vi "LinkamStageController.vi"() -> ()   [LabVIEW 2013]
doc: "The Grab and Save to AVI VI acquires images continuously using the high-level acquisition VIs, displays them in an image control, and saves the images to an AVI file. A grab is appropriate for high-speed applications that process only one image at a time. Use an AVI file to save multiple images to a single file for post-processing or record images.\n\nIMAQ Init initializes the device. IMAQ Grab Setup initializes the grab function and starts capturing images to an internal software buffer. IMAQ Create creates an image buffer IMAQ Grab Acquire copies the internal buffer to Image out, and an image control displays the image on the front panel. IMAQ Close releases resources associated with the acquisition, and IMAQ Dispose frees the image buffer.\n\nIMAQ AVI Create initializes the AVI file, IMAQ AVI WriteFrame adds each image to the AVI file, and IMAQ AVI Close completes writing to the AVI file. Call IMAQ AVI Create for each AVI file created."
uses:
  <vilib>/userdefined/High Color/IMAQdx.ctl
  Mag.ctl
  <vilib>/Instr/_visa.llb/VISA Open Access Mode.ctl
  ImageEnum4GFV.ctl
  RampProgramModel/RampProgramModel.lvclass
  AVI recoder state.ctl
  <vilib>/vision/Avi.llb/IMAQ AVI2 Refnum.ctl
  DateandTime.ctl
  RampProgramModel/RampProgramModel.lvclass/RampProgramModel.ctl
  TextOnImage.ctl
  Ascii Experiment Data.ctl
  RampState.ctl
  <vilib>/Instr/_visa.llb/VISA Configure Serial Port (Instr).vi
  <vilib>/Utility/file.llb/Read From Spreadsheet File (DBL).vi
  <vilib>/Utility/file.llb/Write To Spreadsheet File (string).vi
  <vilib>/vision/driver/NI_Vision_Acquisition_Software.lvlib
  <resource>/objmgr/imaqdx.rc
panel:
  in  "Max(µm)":dbl=55.0 min=0.0 format="%#_g µm"
  in  "Min(µm)":dbl=35.0 min=0.0 format="%#_g µm"
  in  "Enable Droplet Detection":bool=TRUE
  in  "Stop Recording\n@ Temp (°C)":dbl=5.0 format="%#_g °C"
  in  "Start Recording\n@ Temp (°C)":dbl=-2.0 format="%#_g °C"
  in  "Enable\nAutomatic\nRecording":bool=TRUE
  in  "Gain (0-570)":dbl=300.0 min=0.0 max=570.0 step=1.0
  in  "Shutter (1-4095)":dbl=4095.0 min=1.0 max=4095.0 step=1.0
  in  "High Resolution":bool
  in  "Remarks":string
  out "Goal":string
  out "Experiment Name":string
  in  "NewExperiment":bool
  out "File Path":path=path "E:/LINKAM Measurements_Naama"
  in  "Mag":T1
  out "Temp Chart":dbl(graph)
  out "Time Remaining\n(HH:MM:SS)":dbl format="%<%H:%M:%S>t"
  out "Ramp Program Table":string[][](table)
  in  "Clear Table":bool
  in  "Add Entry":bool
  in  "StopProgram":bool
  in  "RunProgram":bool
  in  "PauseProgram":bool
  in  "SaveProgram":bool
  in  "LoadProgram":bool
  in  "Cycles":u32=1 min=1 max=1000 step=1
  out "Cycle No.":u32=1 min=1 max=1000 step=1
  in  "Pump Speed":u8(slide) max=30 step=1 scale=0.0..30.0
  in  "DelayInComm(ms)":u32=50
  out "Video Grabber":bool
  out "Linkam Controller":bool
  out "Ramp Controller":bool
  out "Video Recorder":bool
  in  "Pause":bool caption="Start Cooling/Heating"
  in  "Stop":bool caption="Start Cooling/Heating"
  in  "Record":bool caption="Start Cooling/Heating"
  out "Status":string="Stop"
  in  "TakeRefImage":bool caption="Start Cooling/Heating"
  in  "Time Between Consecutive Frames (sec)":dbl=1.0 caption="Time Between \nConsecutive \nFrames (sec)" min=0.0 max=3600.0 step=0.01 format="%.2g s"
  out "Full avi Path and Name":path=path "Z:/Downloads/data/Test-18_05_2014-15_02_54.avi"
  out "Codec Type":string="Motion JPEG (NI Vision)"
  in  "index 2":i32=4
  in  "error in (no error) 2":errorcluster
  out "Status":string="Stopped"
  out "Repeat Program ind":u32=1 min=1 max=1000 step=1
  in  "error in (no error)":errorcluster
  out "Reference Image":T2(plugin-control)
  in  "Hold Cooling/Heating":bool caption="Start Cooling/Heating"
  in  "Stop Cooling/Heating":bool caption="Start Cooling/Heating"
  in  "Start Cooling/Heating":bool
  in  "Setpoint (°C)":dbl=28.0 min=-100.0 max=50.0 step=0.1 format="%.1g °C"
  in  "Cooling Rate (°C/min)":dbl=1.0 min=0.0 max=20.0 step=0.01 format="%.2g °C/min"
  out "Current Temp (°C)":dbl format="%.1g °C"
  out "Status of Liquied Nitrogen Pump":string="96"
  in  "Max Speed":bool
  in  "LNP mode":bool=TRUE
  out "Error Message":string
  out "Status of Temperature Controller":string
  out "Temp String (C)":string="0.0"
  out "Timer":u32=1002
  out "remaining string":string
  out "read buffer":string
  out "return count":u32
  in  "Session In":T3="cam0"
  out "Image":T2(plugin-control)
  in  "stop":bool
  # "Live Image"
  # "Reference Image"
  # "Select your Camera above"
  # "Linkam Temperature Controller"
  # "Experiment Data"
  # "Video Recorder"
  # "Engines Status"
  # "Status"
  # "Liquid Nitrogen Pump Controller"
  # "Pump Speed"
  # "Video Grabber"
  # "Error Message"
  # "Ramp Table Controller"
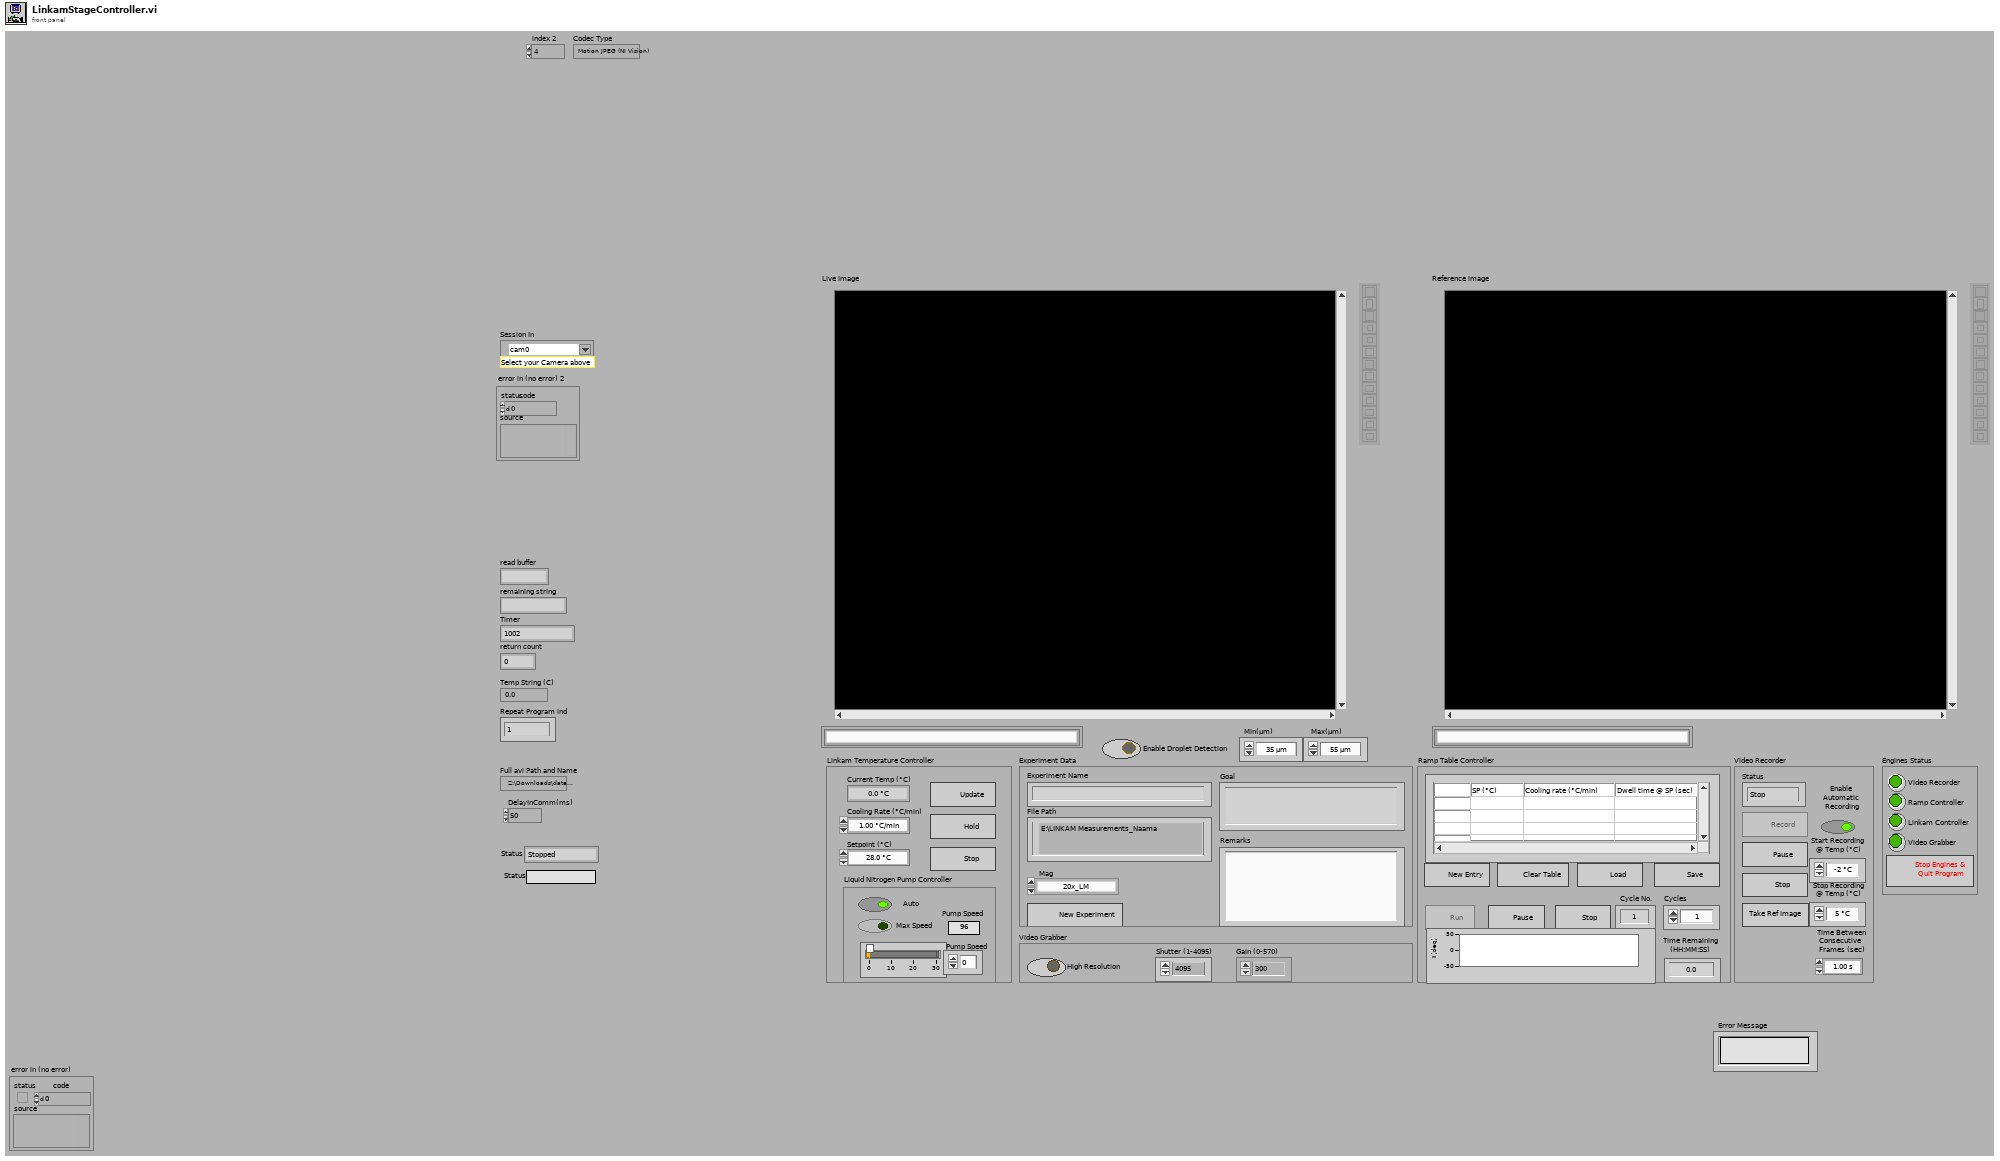
[diagram p1: front panel]
types:
  T1 = typedef "Mag.ctl" = enum16{"20x_LM", "50x_S", "100x_im"}
  T2 = typedef "IMAQ Image.ctl" = refnum<image>
  T3 = typedef "IMAQdx.ctl" = refnum<k21>
  T4 = enum8{"Enabled", "Disabled", "Disabled and Grayed Out"}
  T5 = typedef "DateandTime.ctl" = cluster{"Date and Time":string, "Temp (deg)":string}[]
  T6 = typedef "IMAQ AVI2 Refnum.ctl" = refnum<k20>
  T7 = typedef "AVI recoder state.ctl" = enum16{"Record", "Pause", "Stop", "Init"}
  T8 = typedef "ImageEnum4GFV.ctl" = enum16{"Delete", "Write", "Read", "Init"}
  T9 = typedef "VISA Open Access Mode.ctl" = u32
  T10 = typedef "RampState.ctl" = enum16{"Pause Program", "Heatling/Cooling", "Dwelling @ SP", "Stopped"}
  T11 = typedef "Ascii Experiment Data.ctl" = cluster{"Experiment Name":string, "Goal":string, "Remarks":string, "File Path":string, "Mag":string, "Repeat Program Number":string, "Full avi Path and Name":path, "Ramp Table ":string[][], "Date and Time":T5}
  T12 = cluster{"date/time string":string, "Temp String (C)":string}
  T13 = typedef "TextOnImage.ctl" = cluster{"Status":string, "Experiment Name":string, "Current Temp (C)":string, "Set Point (C)":string, "Cooling Rate (C/min)":string, "Mag":T1}
  T14 = cluster{"Position":cluster{"x":sgl, "y":sgl}, "Angle":sgl, "Scale":sgl, "Score":sgl, "Bounding Box":cluster{"x":sgl, "y":sgl}[]}[]
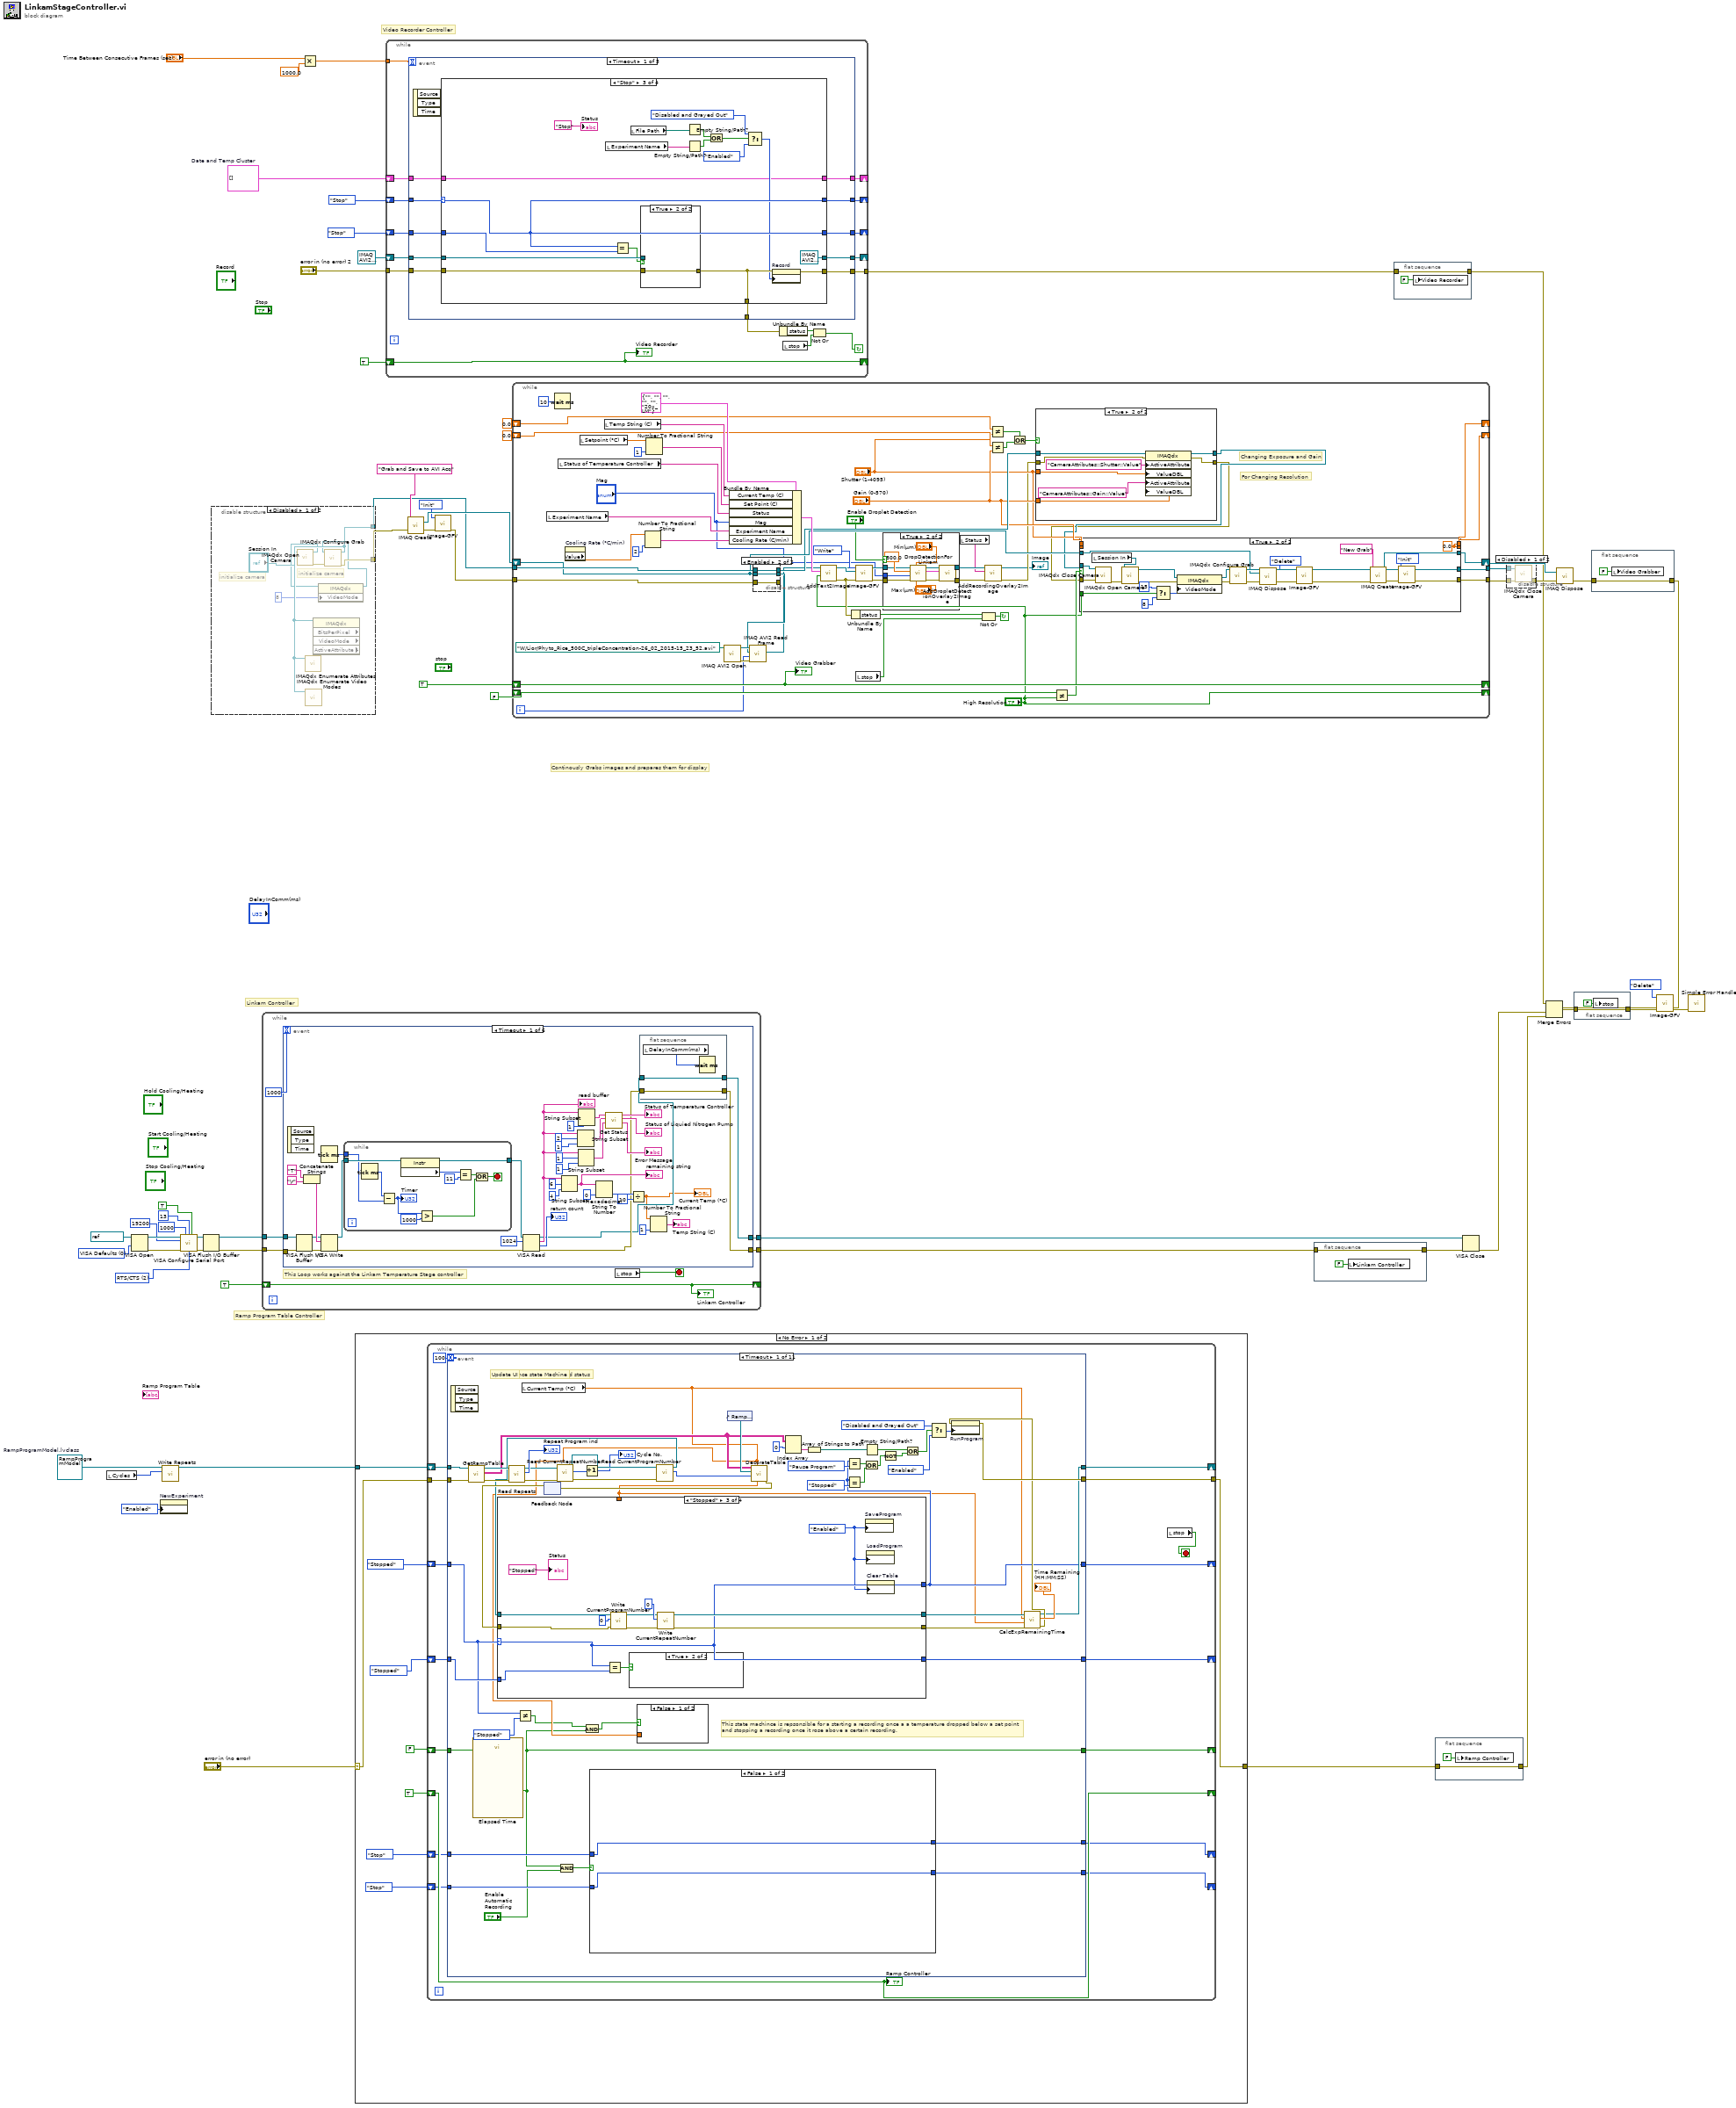
[diagram p0: block diagram]
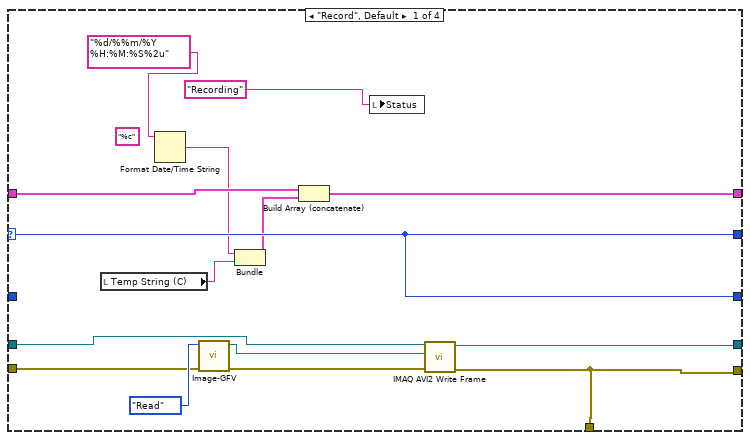
[diagram p4: hidden frame]
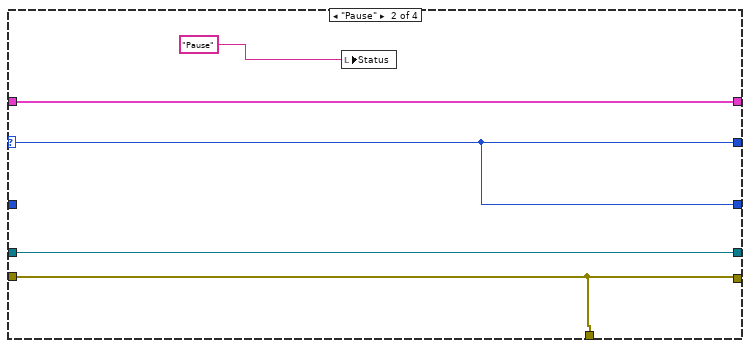
[diagram p5: hidden frame]
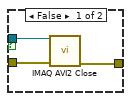
[diagram p6: hidden frame]
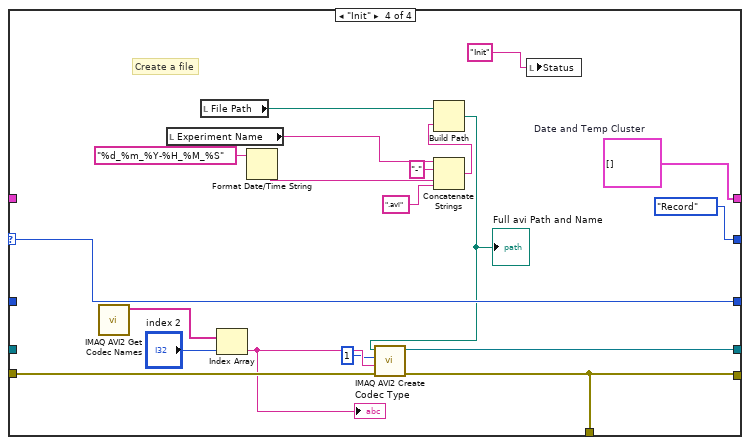
[diagram p7: hidden frame]
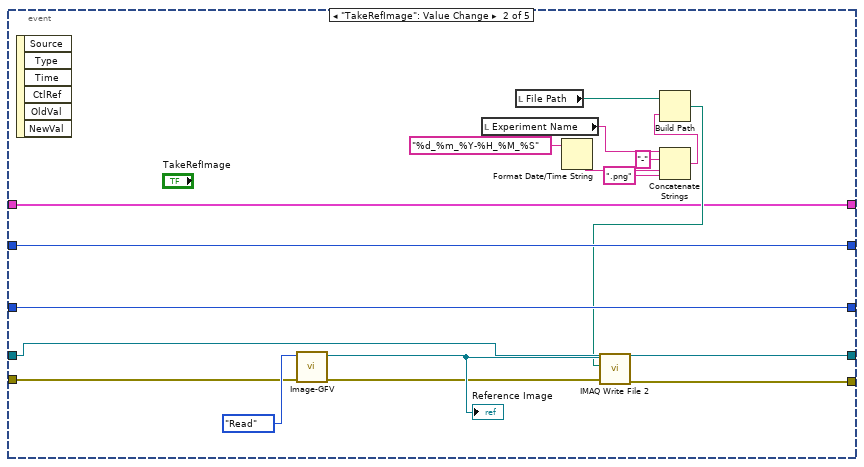
[diagram p8: hidden frame]
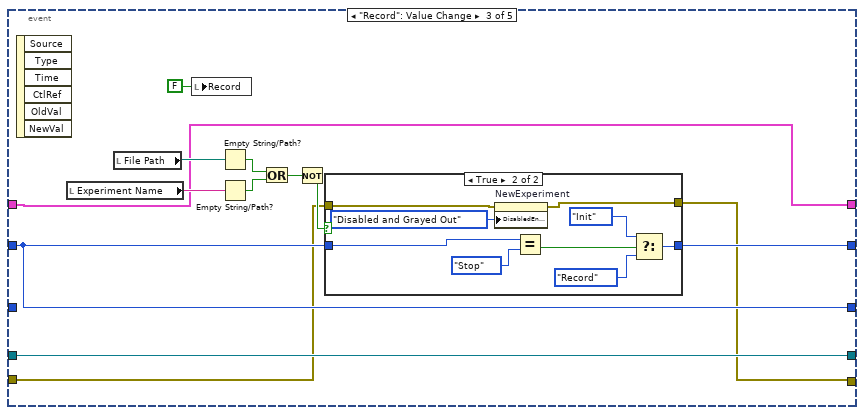
[diagram p9: hidden frame]
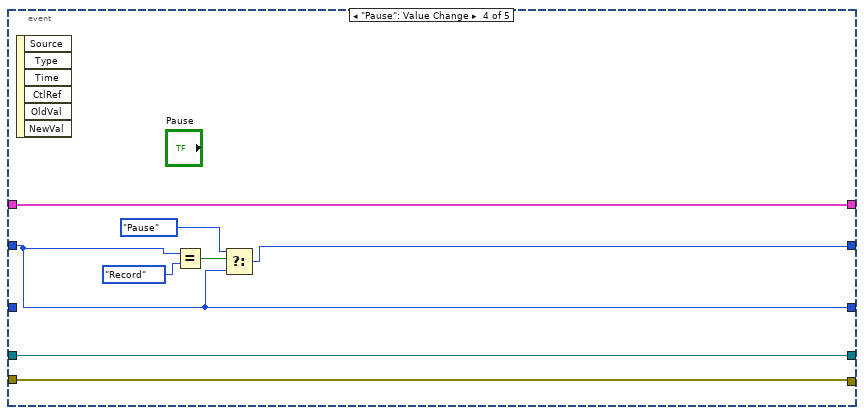
[diagram p11: hidden frame]
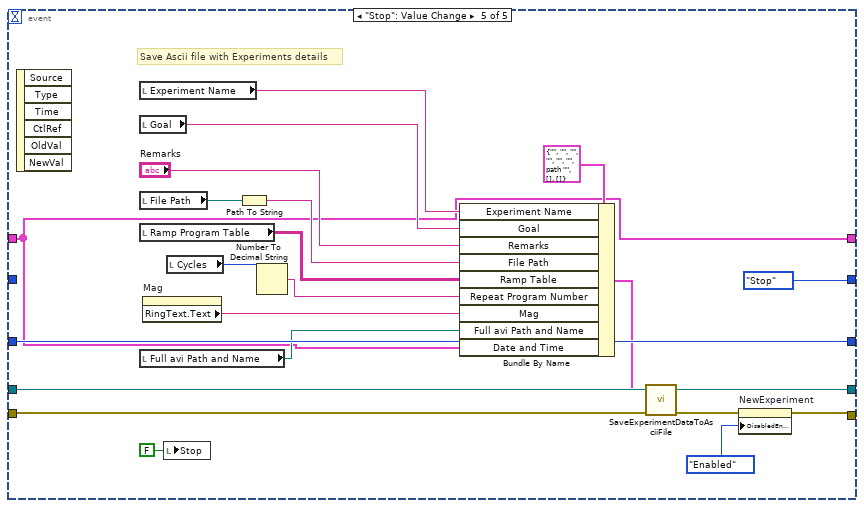
[diagram p12: hidden frame]
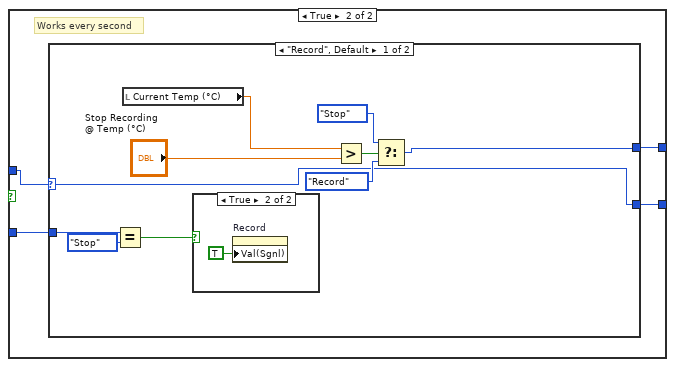
[diagram p13: hidden frame]
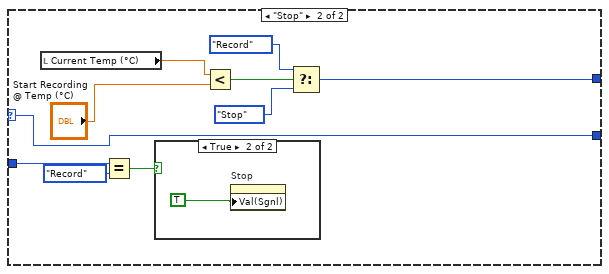
[diagram p15: hidden frame]
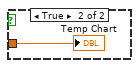
[diagram p17: hidden frame]
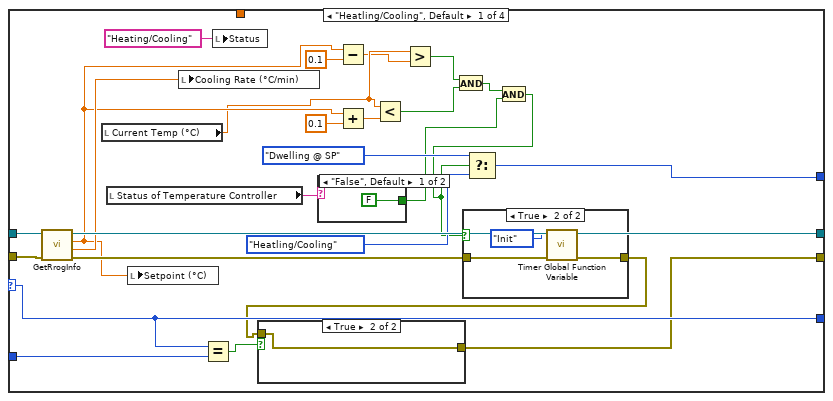
[diagram p18: hidden frame]
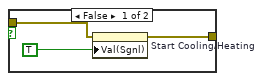
[diagram p19: hidden frame]
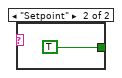
[diagram p20: hidden frame]
diagram:
  w7 = T5 []  # Date and Temp Cluster
  w29 = refnum<class "RampProgramModel.lvclass"> refnum  # RampProgramModel.lvclass
  w48 = T9 0 items=["VISA Defaults"=0, "Exclusive Lock"=1, "Load Configured Settings"=4] ("Access Mode")
  w52 = u16 2 items=["None", "XON/XOFF", "RTS/CTS", "XON/XOFF & RTS/CTS", "DTR/DSR", "XON/XOFF & DTR/DSR"] ("flow control (0:none)")
  # "Linkam Controller"
  # "Video Recorder Controller"
  # "Ramp Program Table Controller"
  # "Continously Grabs images and prepares them for display"
  n1 = local read "Cycles"() -> (w30:u32)
  n2 = VISA Open(access mode=w48, VISA resource name=refnum<visa-resource-name> "COM1") -> (VISA resource name=w55:refnum<visa-resource-name>, error out=w56:errorcluster)  [unwired: 3 in]
  n3 = property on="NewExperiment" class="Bool"("DisabledEnum"=T4."Enabled" ("Disabled")) -> ()  [unwired: 2 in, 2 out]
  n4 = call "Write Repeats.vi"("Repeats"=w30, "RampProgramModel in"=w29) -> ("RampProgramModel out"=w28:refnum<class "RampProgramModel.lvclass">)  [unwired: 8 in, 1 out]
  n5 = call-poly "VISA Configure Serial Port"("VISA resource name"=w55, "timeout (10sec)"=u32 1000, "termination char\n(0xA = '\\n' = LF)"=u8 13 ("termination char\n(0xA = '\\n' = LF)"), "Enable Termination\nChar (T)"=TRUE ("Enable Termination\nChar (T)"), "baud rate (9600)"=u32 19200, "error in (no error)"=w56, "flow control (0:none)"=w52) -> ("VISA resource name out"=w47:refnum<visa-resource-name>, "error out"=w46:errorcluster)  [unwired: 7 in]
  n6 = VISA Flush I/O Buffer(VISA resource name=w47, error in (no error)=w46) -> (VISA resource name out=w45:refnum<visa-resource-name>, error out=w44:errorcluster)  [unwired: 1 in]
  n7 = disable-structure shown="Disabled" {
    disable-tunnel: [w63 _] -> w42
    disable-tunnel: [w62 _] -> w6
    frame Disabled {
      # "initialize camera"
      # "initialize camera"
      n8 = call <vilib>:"IMAQdx Open Camera.vi"("Session In"="Session In") -> ("error out"=w64:errorcluster, "Session Out"=w59:T3)  [unwired: 2 in, 7 out]
      n9 = property class="IMAQdx"(reference=w59, "VideoMode"=u32 8) -> (reference out=w58:T3)  [unwired: 1 in, 1 out]
      n10 = call <vilib>:"IMAQdx Configure Grab.vi"("error in"=w64, "Session In"=w58) -> ("error out"=w63:errorcluster, "Session Out"=w62:T3)  [unwired: 8 out]
      n11 = call <vilib>:"IMAQdx Enumerate Attributes.vi"("Session In"=w62) -> ()  [unwired: 8 in, 3 out]
      n12 = call <vilib>:"IMAQdx Enumerate Video Modes.vi"("Session In"=w62) -> ()  [unwired: 7 in, 4 out]
      n13 = property class="IMAQdx" props=["BitsPerPixel", "VideoMode", "ActiveAttribute"](reference=w62) -> ()  [unwired: 1 in, 5 out]
    }
    frame Enabled {
    }
  }
  n14 = while {
    tunnel: [w71] -> w50
    tunnel: [w70] -> w13
    tunnel: w45 -> [w69]
    tunnel: w44 -> [w68]
    shift-right: [w65] -> _
    shift-left: TRUE -> [w65]
    stop <- w67 stop-if-true
    # "This Loop works against the Linkam Temperature Stage controller"
    n15 = event shown="[0] Timeout" {
      selector: _ -> [_ _ _ _ _ _]
      dyn-events: _ -> [_ _ _ _ _ _]
      timeout: 1000 -> [_ _ _ _ _ _]
      tunnel: [w74 w125 w138 w162 w184 w188] -> w71
      tunnel: [w73 w124 w137 w161 w185 w187] -> w70
      tunnel: w69 -> [w94 w133 w146 w173 w184 w212]
      tunnel: w68 -> [w93 w132 w145 w172 w185 w211]
      event Timeout {
        n16 = event-data() -> ()  [unwired: 1 in, 3 out]
        n17 = VISA Flush I/O Buffer(VISA resource name=w94, error in (no error)=w93) -> (VISA resource name out=w92:refnum<visa-resource-name>, error out=w91:errorcluster)  [unwired: 1 in]
        n18 = Concatenate Strings("T" ("write buffer"), "\r") -> (w95:string)
        n19 = Tick Count (ms)() -> (millisecond timer value=w98:u32)
        n20 = VISA Write(VISA resource name=w92, write buffer=w95, error in (no error)=w91) -> (VISA resource name out=w101:refnum<visa-resource-name>, error out=w99:errorcluster)  [unwired: 1 out]
        n21 = while {
          tunnel: w101 -> [w116]
          tunnel: [w115] -> w100
          tunnel: w98 -> [w114]
          stop <- w117 stop-if-true
          n22 = Tick Count (ms)() -> (millisecond timer value=w121:u32)
          n23 = Subtract(x=w121, y=w114) -> (x-y=w113:u32)
          "Timer" <- w113
          n24 = property class="Instr"(reference=w116) -> (reference out=w115:refnum<visa-resource-name>, "Serial Settings:Number of Bytes at Serial Port"=w123:u32)  [unwired: 1 in, 1 out]
          n25 = Greater?(x=w113, y=u32 1000) -> (0:w118:bool)
          n26 = Equal?(x=w123, y=u32 11) -> (x = y?=w119:bool)
          n27 = Or(x=w119, y=w118) -> (x .or. y?=w117:bool)
        }
        n28 = VISA Read(VISA resource name=w100, byte count=u32 1024, error in (no error)=w99) -> (VISA resource name out=w75:refnum<visa-resource-name>, read buffer=w79:string, return count=→"return count":u32, error out=w76:errorcluster)
        "read buffer" <- w79
        n29 = String Subset(string=w79, offset (0)=6, length (rest)=4 ("length (rest)")) -> (substring=w104:string)
        "remaining string" <- w104
        n30 = String Subset(string=w79, offset (0)=2, length (rest)=1 ("length (rest)")) -> (substring=w83:string)
        n31 = String Subset(string=w79, offset (0)=1, length (rest)=1 ("length (rest)")) -> (substring=w78:string)
        n32 = String Subset(string=w79, length (rest)=1 ("length (rest)")) -> (substring=w87:string)  [unwired: 1 in]
        n33 = Hexadecimal String To Number(string=w104, default (0uL)=i16 0 ("default (0 U32)")) -> (number=w103:i16)  [unwired: 1 in, 1 out]
        n34 = call "Get Status.vi"("Error message input"=w78, "Input Pump Status string"=w83, "Input Status String"=w87) -> ("Error message string"=→"Error Message":string, "Output Pump Status"=→"Status of Liquied Nitrogen Pump":string, "Output Status String"=→"Status of Temperature Controller":string)  [unwired: 6 in]
        n35 = Divide(x=w103, y=i16 10) -> (x/y=w72:dbl)
        "Current Temp (°C)" <- w72
        n36 = flat-sequence {
          tunnel: w76 -> [w112]
          tunnel: [w112] -> w73
          tunnel: w75 -> [w111]
          tunnel: [w111] -> w74
          frame #0 {
            n37 = local read "DelayInComm(ms)"() -> (w110:u32)
            n38 = Wait (ms)(milliseconds to wait=w110) -> ()  [unwired: 1 out]
          }
        }
        n39 = Number To Fractional String(number=w72, precision (6)=i16 1) -> (F-format string=→"Temp String (C)":string)  [unwired: 2 in]
      }
      event "Stop Cooling/Heating": Value Change {
        n40 = event-data() -> ()  [unwired: 1 in, 6 out]
        n41 = Concatenate Strings("E" ("write buffer"), "\r") -> (w129:string)
        n42 = VISA Write(VISA resource name=w133, write buffer=w129, error in (no error)=w132) -> (VISA resource name out=w127:refnum<visa-resource-name>, error out=w126:errorcluster)  [unwired: 1 out]
        n43 = flat-sequence {
          tunnel: w126 -> [w136]
          tunnel: [w136] -> w124
          tunnel: w127 -> [w135]
          tunnel: [w135] -> w125
          frame #0 {
            n44 = local read "DelayInComm(ms)"() -> (w134:u32)
            n45 = Wait (ms)(milliseconds to wait=w134) -> ()  [unwired: 1 out]
          }
        }
        n46 = local write "Stop Cooling/Heating"(FALSE ("Stop Cooling/Heating")) -> ()
      }
      event "Hold Cooling/Heating": Value Change {
        n47 = event-data() -> ()  [unwired: 1 in, 6 out]
        n48 = Concatenate Strings("OCR" ("write buffer"), "\r") -> (w142:string)
        n49 = VISA Write(VISA resource name=w146, write buffer=w142, error in (no error)=w145) -> (VISA resource name out=w140:refnum<visa-resource-name>, error out=w139:errorcluster)  [unwired: 1 out]
        n50 = local write "Hold Cooling/Heating"(FALSE ("Hold Cooling/Heating")) -> ()
        n51 = flat-sequence {
          tunnel: w139 -> [w149]
          tunnel: [w149] -> w137
          tunnel: w140 -> [w148]
          tunnel: [w148] -> w138
          frame #0 {
            n52 = local read "DelayInComm(ms)"() -> (w147:u32)
            n53 = Wait (ms)(milliseconds to wait=w147) -> ()  [unwired: 1 out]
          }
        }
      }
      event "LNP mode", "Pump Speed": Value Change {
        n54 = event-data() -> ()  [unwired: 1 in, 6 out]
        n55 = Select(t="Pa0", s="LNP mode", f="Pm0") -> (s? t:f=w168:string)
        n56 = Concatenate Strings(w168, "\r") -> (w170:string)
        n57 = VISA Write(VISA resource name=w173, write buffer=w170, error in (no error)=w172) -> (VISA resource name out=w160:refnum<visa-resource-name>, error out=w159:errorcluster)  [unwired: 1 out]
        n58 = flat-sequence {
          tunnel: w159 -> [w176]
          tunnel: [w176] -> w158
          tunnel: w160 -> [w175]
          tunnel: [w175] -> w157
          frame #0 {
            n59 = local read "DelayInComm(ms)"() -> (w174:u32)
            n60 = Wait (ms)(milliseconds to wait=w174) -> ()  [unwired: 1 out]
          }
        }
        n61 = Add(x="Pump Speed", y=u8 48) -> (x+y=w154:u8)
        n62 = Type Cast(x=w154) -> (*(type *) &x=w152:string)  [unwired: 1 out]
        n63 = Concatenate Strings("P" ("string"), w152) -> (w151:string)
        n64 = Concatenate Strings(w151, "\r") -> (w165:string)
        n65 = VISA Write(VISA resource name=w157, write buffer=w165, error in (no error)=w158) -> (VISA resource name out=w164:refnum<visa-resource-name>, error out=w163:errorcluster)  [unwired: 1 out]
        n66 = flat-sequence {
          tunnel: w163 -> [w179]
          tunnel: [w179] -> w161
          tunnel: w164 -> [w178]
          tunnel: [w178] -> w162
          frame #0 {
            n67 = local read "DelayInComm(ms)"() -> (w177:u32)
            n68 = Wait (ms)(milliseconds to wait=w177) -> ()  [unwired: 1 out]
          }
        }
      }
      event "Max Speed": Value Change {
        n69 = event-data() -> ()  [unwired: 1 in, 6 out]
        n70 = Select(t=u8 30 ("f"), s="Max Speed", f=u8 0) -> (s? t:f=w182:u8)
        n71 = property on="Pump Speed" class="Slide (strict)"("Val(Sgnl)"=w182) -> ()  [unwired: 2 in, 2 out]
      }
      event "Start Cooling/Heating": Value Change {
        # "Caused to max speed at every update"
        n72 = event-data() -> ()  [unwired: 1 in, 6 out]
        n73 = Multiply(x="Cooling Rate (°C/min)", y=u16 100) -> (x*y=w201:dbl)
        n74 = To Long Integer(number=w201) -> (32bit integer=w200:i32)
        n75 = Number To Decimal String(number=w200) -> (decimal integer string=w213:string)  [unwired: 1 in]
        n76 = property on="LNP mode" class="Bool (strict)"() -> ("Value"=w186:bool)  [unwired: 2 in, 2 out]
        n77 = Concatenate Strings("R1" ("write buffer"), w213, "\r") -> (w210:string)
        n78 = VISA Write(VISA resource name=w212, write buffer=w210, error in (no error)=w211) -> (VISA resource name out=w197:refnum<visa-resource-name>, error out=w198:errorcluster)  [unwired: 1 out]
        n79 = case shown="False" w186 {
          frame False {
            n80 = property on="LNP mode" class="Bool (strict)"("Val(Sgnl)"=TRUE ("LNP mode")) -> ()  [unwired: 2 in, 2 out]
          }
          frame True {
          }
        }
        n81 = flat-sequence {
          tunnel: w198 -> [w229]
          tunnel: [w229] -> w195
          tunnel: w197 -> [w228]
          tunnel: [w228] -> w196
          frame #0 {
            n82 = local read "DelayInComm(ms)"() -> (w227:u32)
            n83 = Wait (ms)(milliseconds to wait=w227) -> ()  [unwired: 1 out]
          }
        }
        n84 = local write "Start Cooling/Heating"(FALSE ("Start Cooling/Heating")) -> ()
        n85 = Multiply(x="Setpoint (°C)", y=u16 10) -> (x*y=w208:dbl)
        n86 = Number To Decimal String(number=w208) -> (decimal integer string=w209:string)  [unwired: 1 in]
        n87 = Concatenate Strings("L1" ("write buffer"), w209, "\r") -> (w203:string)
        n88 = VISA Write(VISA resource name=w196, write buffer=w203, error in (no error)=w195) -> (VISA resource name out=w194:refnum<visa-resource-name>, error out=w193:errorcluster)  [unwired: 1 out]
        n89 = flat-sequence {
          tunnel: w193 -> [w226]
          tunnel: [w226] -> w191
          tunnel: w194 -> [w225]
          tunnel: [w225] -> w192
          frame #0 {
            n90 = local read "DelayInComm(ms)"() -> (w224:u32)
            n91 = Wait (ms)(milliseconds to wait=w224) -> ()  [unwired: 1 out]
          }
        }
        n92 = flat-sequence {
          tunnel: w189 -> [w223]
          tunnel: [w223] -> w187
          tunnel: w190 -> [w222]
          tunnel: [w222] -> w188
          frame #0 {
            n93 = local read "DelayInComm(ms)"() -> (w221:u32)
            n94 = Wait (ms)(milliseconds to wait=w221) -> ()  [unwired: 1 out]
          }
        }
        n95 = Concatenate Strings("S" ("write buffer"), "\r") -> (w217:string)
        n96 = VISA Write(VISA resource name=w192, write buffer=w217, error in (no error)=w191) -> (VISA resource name out=w190:refnum<visa-resource-name>, error out=w189:errorcluster)  [unwired: 1 out]
      }
    }
    n97 = local read "stop"() -> (w67:bool)
    "Linkam Controller" <- w65
  }
  n98 = Multiply(x="Time Between Consecutive Frames (sec)", y=1000.0) -> (x*y=w25:dbl)
  n99 = case shown="No Error" "error in (no error)" {
    selector: "error in (no error)" -> [w238 w547]
    tunnel: [w237 w547] -> w15
    tunnel: w28 -> [w236 _]
    frame No Error {
      n100 = while {
        tunnel: w238 -> [w255]
        tunnel: [w254] -> w237
        shift-right: [w252] -> _
        shift-left: w236 -> [w253]
        shift-right: [w249] -> _
        shift-left: RampState."Stopped" ("State") -> [w250]
        shift-right: [w247] -> _
        shift-left: RampState."Stopped" ("State") -> [w246]
        shift-right: [w245] -> _
        shift-left: TRUE -> [w245]
        shift-right: [w243] -> _
        shift-left: FALSE -> [w244]
        shift-right: [w240] -> _
        shift-left: AVI_recoder_state."Stop" -> [w242]
        shift-right: [w239] -> _
        shift-left: AVI_recoder_state."Stop" -> [w241]
        stop <- w248 stop-if-true
        n101 = event shown="[0] Timeout" {
          selector: _ -> [_ _ _ _ _ _ _ _ _ _ _]
          dyn-events: _ -> [_ _ _ _ _ _ _ _ _ _ _]
          timeout: u32 100 ("milliseconds to wait") -> [_ _ _ _ _ _ _ _ _ _ _]
          tunnel: w255 -> [w309 w456 w468 w477 w485 w492 w498 w507 w514 w527 w544]
          tunnel: [w292 w455 w468 w476 w485 w490 w498 w507 w514 w522 w543] -> w254
          tunnel: w253 -> [w308 w459 w469 w478 w484 w493 w499 w508 w513 w520 w545]
          tunnel: [w282 w459 w469 w475 w483 w491 w499 w508 w513 w521 w542] -> w252
          tunnel: w250 -> [w269 w458 w467 w473 w481 w488 _ _ _ w519 w546]
          tunnel: [w277 w458 w467 w473 w481 w488 RampState."Pause Program" ("State") RampState."Heatling/Cooling" ("State") RampState."Stopped" ("State") w519 w546] -> w249
          tunnel: [w300 w457 w466 w473 w481 w488 w496 w504 w512 w518 w540] -> w247
          tunnel: w246 -> [w299 w457 w466 _ _ _ w496 w504 w512 w518 w540]
          tunnel: w244 -> [w265 _ _ _ _ _ _ _ _ _ _]
          tunnel: [w256 _ _ _ _ _ _ _ _ _ _] -> w243
          tunnel: w242 -> [w262 w450 w465 w472 w480 w487 w495 w501 w511 w517 w539]
          tunnel: w241 -> [w261 w449 w464 w471 w479 w486 w494 w500 w510 w516 w538]
          tunnel: [w260 w450 w465 w472 w480 w487 w495 w501 w511 w517 w539] -> w240
          tunnel: [w257 w449 w464 w471 w479 w486 w494 w500 w510 w516 w538] -> w239
          event Timeout {
            # "This state machince is repsonsible for a starting a recording once a a temperature dropped below a set point \nand stopping a recording once it rose above a certain recording."
            # "Read Current Temperture and status"
            # "And advance state Machine"
            # "Update UI"
            n102 = event-data() -> ()  [unwired: 1 in, 3 out]
            n103 = call "GetRampTable.vi"("error in (no error)"=w309, "RampProgramModel in"=w308) -> ("error out"=w305:errorcluster, "RampTable"=w298:string[][], "RampProgramModel out"=w307:refnum<class "RampProgramModel.lvclass">)  [unwired: 7 in]
            n104 = call "Elapsed Time"("Reset"=w265) -> ("Time has Elapsed"=w256:bool)  [unwired: 11 in, 7 out]
            n105 = call "Read Repeats.vi"("error in (no error)"=w305, "RampProgramModel in"=w307) -> ("error out"=w303:errorcluster, "Repeats"=→"Repeat Program ind":u32, "RampProgramModel out"=w304:refnum<class "RampProgramModel.lvclass">)  [unwired: 7 in]
            n106 = Not Equal?(x=w269, y=RampState."Stopped" ("State")) -> (x != y?=w263:bool)
            n107 = local read "Current Temp (°C)"() -> (w264:dbl)
            n108 = feedback #1() -> (w290:errorcluster)  [unwired: 1 in]
            n109 = call "Read CurrentRepeatNumber.vi"("error in (no error)"=w303, "RampProgramModel in"=w304) -> ("error out"=w287:errorcluster, "CurrentRepeatNumber"=w271:u32, "RampProgramModel out"=w288:refnum<class "RampProgramModel.lvclass">)  [unwired: 7 in]
            n110 = And(x=w256, y="Enable\nAutomatic\nRecording") -> (x .and. y?=w258:bool)
            n111 = Increment(x=w271) -> (x+1=→"Cycle No.":u32)
            n112 = And(x=w263, y=w256) -> (x .and. y?=w266:bool)
            n113 = case shown="False" w258 {
              tunnel: w262 -> [w311 w315]
              tunnel: w261 -> [w310 w314]
              tunnel: [w311 w313] -> w260
              tunnel: [w310 w312] -> w257
              frame False {
              }
              frame True {
                # "Works every second"
                n114 = case shown="\"Record\", Default" w315 {
                  selector: w315 -> [w317 w328]
                  tunnel: w314 -> [w325 w331]
                  tunnel: [w319 w333] -> w313
                  tunnel: [w317 w328] -> w312
                  frame "Record", Default {
                    n115 = Equal?(x=w325, y=AVI_recoder_state."Stop") -> (x = y?=w323:bool)
                    n116 = local read "Current Temp (°C)"() -> (w316:dbl)
                    n117 = case shown="True" w323 {
                      frame False {
                      }
                      frame True {
                        n118 = property on="Record" class="Bool (strict)"("Val(Sgnl)"=TRUE ("Value (Signaling)")) -> ()  [unwired: 2 in, 2 out]
                      }
                    }
                    n119 = Greater?(x=w316, y="Stop Recording\n@ Temp (°C)") -> (0:w322:bool)
                    n120 = Select(t=AVI_recoder_state."Stop" ("y"), s=w322, f=AVI_recoder_state."Record" ("y")) -> (s? t:f=w319:T7)
                  }
                  frame "Stop" {
                    n121 = local read "Current Temp (°C)"() -> (w327:dbl)
                    n122 = Equal?(x=w331, y=AVI_recoder_state."Record") -> (x = y?=w330:bool)
                    n123 = case shown="True" w330 {
                      frame False {
                      }
                      frame True {
                        n124 = property on="Stop" class="Bool (strict)"("Val(Sgnl)"=TRUE ("Value (Signaling)")) -> ()  [unwired: 2 in, 2 out]
                      }
                    }
                    n125 = Less?(x=w327, y="Start Recording\n@ Temp (°C)") -> (x < y?=w336:bool)
                    n126 = Select(t=AVI_recoder_state."Record", s=w336, f=AVI_recoder_state."Stop") -> (s? t:f=w333:T7)
                  }
                }
              }
            }
            n127 = case shown="False" w266 {
              tunnel: w264 -> [_ w338]
              frame False {
              }
              frame True {
                "Temp Chart" <- w338
              }
            }
            n128 = call "Read CurrentProgramNumber.vi"("error in (no error)"=w287, "RampProgramModel in"=w288) -> ("CurrentProgramNumber"=w301:u32, "RampProgramModel out"=w285:refnum<class "RampProgramModel.lvclass">)  [unwired: 7 in, 1 out]
            n129 = case shown="\"Stopped\"" w269 {
              selector: w269 -> [w354 w376 w432 w444]
              tunnel: [w359 w383 w432 w444] -> w277
              tunnel: w285 -> [w363 w387 w439 w446]
              tunnel: [w362 w380 w433 w446] -> w286
              tunnel: [w340 w379 w434 w442] -> w284
              tunnel: [_ w378 _ _] -> w267
              tunnel: [w354 w377 w432 w444] -> w300
              tunnel: w299 -> [w355 _ w431 w445]
              tunnel: w290 -> [w339 w375 w429 w442]
              frame "Heatling/Cooling", Default {
                n130 = call "GetRrogInfo.vi"("error in (no error)"=w339, "RampProgramModel in"=w363) -> ("error out"=w358:errorcluster, "Cooling rate (°C/min)"=w357:dbl, "SP (°C)"=w350:dbl, "RampProgramModel out"=w362:refnum<class "RampProgramModel.lvclass">)  [unwired: 5 in, 1 out]
                n131 = local read "Current Temp (°C)"() -> (w348:dbl)
                n132 = local read "Status of Temperature Controller"() -> (w356:string)
                n133 = local write "Setpoint (°C)"(w350) -> ()
                n134 = local write "Cooling Rate (°C/min)"(w357) -> ()
                n135 = Equal?(x=w354, y=w355) -> (x = y?=w353:bool)
                n136 = local write "Status"("Heating/Cooling" ("Status")) -> ()
                n137 = case shown="\"False\", Default" w356 {
                  tunnel: [FALSE TRUE] -> w343
                  frame "False", Default {
                  }
                  frame "Setpoint" {
                  }
                }
                n138 = Subtract(x=w350, y=0.1) -> (x-y=w347:dbl)
                n139 = Add(x=w350, y=0.1) -> (x+y=w349:dbl)
                n140 = Less?(x=w348, y=w349) -> (x < y?=w345:bool)
                n141 = Greater?(x=w348, y=w347) -> (0:w346:bool)
                n142 = And(x=w346, y=w345) -> (x .and. y?=w344:bool)
                n143 = And(x=w344, y=w343) -> (x .and. y?=w342:bool)
                n144 = case shown="True" w342 {
                  tunnel: w358 -> [w371 w373]
                  tunnel: [w371 w372] -> w341
                  frame False {
                  }
                  frame True {
                    n145 = call "Timer Global Function Variable.vi"("error in (no error)"=w373, "Enum"=enum16{"Init", "Read", "Set"}."Init") -> ("error out"=w372:errorcluster)  [unwired: 7 in, 2 out]
                  }
                }
                n146 = case shown="True" w353 {
                  tunnel: w341 -> [w366 w368]
                  tunnel: [w365 w368] -> w340
                  frame False {
                    n147 = property on="Start Cooling/Heating" class="Bool (strict)"(error in=w366, "Val(Sgnl)"=TRUE) -> (error out=w365:errorcluster)  [unwired: 1 in, 1 out]
                  }
                  frame True {
                  }
                }
                n148 = Select(t=RampState."Dwelling @ SP" ("State"), s=w342, f=RampState."Heatling/Cooling" ("State")) -> (s? t:f=w359:T10)
              }
              frame "Dwelling @ SP" {
                n149 = call "GetRrogInfo.vi"("error in (no error)"=w375, "RampProgramModel in"=w387) -> ("error out"=w381:errorcluster, "RampProgramModel out"=w382:refnum<class "RampProgramModel.lvclass">, "Dwell Time @ SP (sec)"=w385:u32)  [unwired: 5 in, 2 out]
                n150 = local write "Status"("Dwelling" ("Status")) -> ()
                n151 = call "Timer Global Function Variable.vi"("Enum"=enum16{"Init", "Read", "Set"}."Read") -> ("Time Elapsed"=w378:dbl)  [unwired: 8 in, 2 out]
                n152 = Greater Or Equal?(x=w378, y=w385) -> (x >= y?=w384:bool)
                n153 = case shown="True" w384 {
                  tunnel: [RampState."Dwelling @ SP" ("State") w397] -> w383
                  tunnel: w382 -> [w391 w402]
                  tunnel: w381 -> [w390 w401]
                  tunnel: [w391 w396] -> w380
                  tunnel: [w390 w395] -> w379
                  tunnel: [w389 w394] -> w377
                  tunnel: w376 -> [w389 w393]
                  frame False {
                  }
                  frame True {
                    n154 = call "AdvanceRampProg.vi"("error in (no error)"=w401, "RampProgramModel in"=w402) -> ("error out"=w398:errorcluster, "EndOfPrograms"=w400:bool, "RampProgramModel out"=w399:refnum<class "RampProgramModel.lvclass">)  [unwired: 7 in]
                    n155 = case shown="True" w400 {
                      tunnel: w399 -> [w404 w416]
                      tunnel: w398 -> [w405 w415]
                      tunnel: [RampState."Heatling/Cooling" ("State") w411] -> w397
                      tunnel: [w404 w410] -> w396
                      tunnel: [w405 w409] -> w395
                      tunnel: [w403 w408] -> w394
                      tunnel: w393 -> [w403 w407]
                      frame False {
                      }
                      frame True {
                        n156 = call "AdvanceCurrentRepeat.vi"("error in (no error)"=w415, "RampProgramModel in"=w416) -> ("error out"=w412:errorcluster, "EndOfRepeats"=w414:bool, "RampProgramModel out"=w413:refnum<class "RampProgramModel.lvclass">)  [unwired: 7 in]
                        n157 = case shown="True" w414 {
                          tunnel: w413 -> [w421 w425]
                          tunnel: w412 -> [w420 w426]
                          tunnel: [RampState."Heatling/Cooling" ("State") RampState."Stopped" ("State")] -> w411
                          tunnel: [w418 w425] -> w410
                          tunnel: [w419 w426] -> w409
                          tunnel: [w417 w424] -> w408
                          tunnel: w407 -> [w417 w424]
                          frame False {
                            n158 = call "Write CurrentProgramNumber.vi"("error in (no error)"=w420, "CurrentProgramNumber"=u32 0, "RampProgramModel in"=w421) -> ("error out"=w419:errorcluster, "RampProgramModel out"=w418:refnum<class "RampProgramModel.lvclass">)  [unwired: 7 in]
                          }
                          frame True {
                          }
                        }
                      }
                    }
                  }
                }
              }
              frame "Stopped" {
                w428 = T4."Enabled" ("Disabled")
                n159 = Equal?(x=w432, y=w431) -> (x = y?=w430:bool)
                n160 = call "Write CurrentProgramNumber.vi"("error in (no error)"=w429, "CurrentProgramNumber"=u32 0, "RampProgramModel in"=w439) -> ("error out"=w435:errorcluster, "RampProgramModel out"=w436:refnum<class "RampProgramModel.lvclass">)  [unwired: 7 in]
                n161 = case shown="True" w430 {
                  frame False {
                    n162 = property on="Stop Cooling/Heating" class="Bool (strict)"("Val(Sgnl)"=TRUE ("Value (Signaling)")) -> ()  [unwired: 2 in, 2 out]
                  }
                  frame True {
                  }
                }
                n163 = call "Write CurrentRepeatNumber.vi"("error in (no error)"=w435, "CurrentRepeatNumber"=u32 0, "RampProgramModel in"=w436) -> ("error out"=w434:errorcluster, "RampProgramModel out"=w433:refnum<class "RampProgramModel.lvclass">)  [unwired: 7 in]
                n164 = property on="SaveProgram" class="Bool"("DisabledEnum"=w428) -> ()  [unwired: 2 in, 2 out]
                n165 = property on="LoadProgram" class="Bool"("DisabledEnum"=w428) -> ()  [unwired: 2 in, 2 out]
                n166 = property on="Clear Table" class="Bool"("DisabledEnum"=w428) -> ()  [unwired: 2 in, 2 out]
                "Status" <- "Stopped" ("Status")
              }
              frame "Pause Program" {
                # "Send the hold command to the controller"
                n167 = Equal?(x=w444, y=w445) -> (x = y?=w443:bool)
                n168 = case shown="False" w443 {
                  frame False {
                    n169 = property on="Hold Cooling/Heating" class="Bool (strict)"("Val(Sgnl)"=TRUE ("Value (Signaling)")) -> ()  [unwired: 2 in, 2 out]
                  }
                  frame True {
                  }
                }
                n170 = local write "Status"("Pause" ("Status")) -> ()
              }
            }
            n171 = control-ref of="Ramp Program Table"() -> (w302:refnum<vi>)
            n172 = call "DecorateTable.vi"("Elapsed Time"=w267, "Current Temperature"=w264, "Current Program"=w301, "Tbl Refnum"=w302, "RampTable"=w298) -> ("error out"=w291:errorcluster)  [unwired: 6 in]
            n173 = feedback-in #1(w291) -> ()
            n174 = Index Array(array=w298, index (row)=0) -> (element=w296:string[])  [unwired: 1 in]
            n175 = Array of Strings to Path(0:w296) -> (2:w295:path)  [unwired: 1 in]
            n176 = Equal?(x=w277, y=RampState."Pause Program" ("State")) -> (x = y?=w276:bool)
            n177 = Equal?(x=w277, y=RampState."Stopped" ("State")) -> (x = y?=w279:bool)
            n178 = Empty String/Path?(string/path=w295) -> (empty?=w275:bool)
            n179 = Or(x=w276, y=w279) -> (x .or. y?=w273:bool)
            n180 = Not(x=w273) -> (.not. x?=w272:bool)
            n181 = Or(x=w275, y=w272) -> (x .or. y?=w274:bool)
            n182 = Select(t=T4."Disabled and Grayed Out" ("Disabled"), s=w274, f=T4."Enabled" ("Disabled")) -> (s? t:f=w293:T4)
            n183 = call "CalcExpRemainingTime.vi"("error in (no error)"=w284, "Current Dwell Time"=w267, "Current Temperature"=w264, "RampProgramModel in"=w286) -> ("error out"=w283:errorcluster, "RemainExpTime(sec)"=→"Time Remaining\n(HH:MM:SS)":dbl, "RampProgramModel out"=w282:refnum<class "RampProgramModel.lvclass">)  [unwired: 5 in]
            n184 = property on="RunProgram" class="Bool"(error in=w283, "DisabledEnum"=w293) -> (error out=w292:errorcluster)  [unwired: 1 in, 1 out]
          }
          event "NewExperiment": Value Change {
            n185 = event-data() -> ()  [unwired: 1 in, 6 out]
            n186 = call "NewExperimentDialog.vi"("error in (no error)"=w456) -> ("error out"=w455:errorcluster, "Goal 2"=w452:string, "File Path 2"=w451:path, "Experiment Name 2"=w453:string, "Add Entry Pressed?"=w454:bool)  [unwired: 6 in]
            n187 = case shown="True" w454 {
              tunnel: w453 -> [_ w462]
              tunnel: w452 -> [_ w461]
              tunnel: w451 -> [_ w460]
              frame False {
              }
              frame True {
                "Experiment Name" <- w462
                "Goal" <- w461
                "File Path" <- w460
              }
            }
          }
          event "Enable\nAutomatic\nRecording": Value Change {
            n188 = event-data() -> ("NewVal"=w463:bool)  [unwired: 1 in, 5 out]
            n189 = case shown="True" w463 {
              frame False {
              }
              frame True {
                n190 = property on="Stop" class="Bool (strict)"("Val(Sgnl)"=TRUE ("Value (Signaling)")) -> ()  [unwired: 2 in, 2 out]
              }
            }
          }
          event "Cycles": Value Change {
            n191 = event-data() -> ()  [unwired: 1 in, 6 out]
            n192 = call "Write Repeats.vi"("error in (no error)"=w477, "Repeats"="Cycles", "RampProgramModel in"=w478) -> ("error out"=w476:errorcluster, "RampProgramModel out"=w475:refnum<class "RampProgramModel.lvclass">)  [unwired: 7 in]
          }
          event "LoadProgram": Value Change {
            n193 = event-data() -> ()  [unwired: 1 in, 6 out]
            n194 = call-poly <vilib>:"Read From Spreadsheet File.vi"() -> ("all rows"=w482:dbl[][])  [unwired: 7 in, 4 out]
            n195 = call "WriteRampTable.vi"("RampFromFile"=w482, "RampProgramModel in"=w484) -> ("RampProgramModel out"=w483:refnum<class "RampProgramModel.lvclass">)  [unwired: 8 in, 1 out]
          }
          event "SaveProgram": Value Change {
            n196 = event-data() -> ()  [unwired: 1 in, 6 out]
            n197 = call "GetRampTable.vi"("error in (no error)"=w492, "RampProgramModel in"=w493) -> ("error out"=w490:errorcluster, "RampTable"=w489:string[][], "RampProgramModel out"=w491:refnum<class "RampProgramModel.lvclass">)  [unwired: 7 in]
            n198 = call-poly <vilib>:"Write To Spreadsheet File.vi"("2D data"=w489) -> ()  [unwired: 7 in, 1 out]
          }
          event "PauseProgram": Value Change {
            n199 = event-data() -> ()  [unwired: 1 in, 6 out]
          }
          event "RunProgram": Value Change {
            w505 = T4."Disabled and Grayed Out" ("Disabled")
            n200 = event-data() -> ()  [unwired: 1 in, 6 out]
            n201 = Not Equal?(x=w504, y=RampState."Pause Program" ("State")) -> (x != y?=w502:bool)
            n202 = property on="SaveProgram" class="Bool"("DisabledEnum"=w505) -> ()  [unwired: 2 in, 2 out]
            n203 = property on="LoadProgram" class="Bool"("DisabledEnum"=w505) -> ()  [unwired: 2 in, 2 out]
            n204 = property on="Clear Table" class="Bool"("DisabledEnum"=w505) -> ()  [unwired: 2 in, 2 out]
            n205 = property on="RunProgram" class="Bool"("DisabledEnum"=w505) -> ()  [unwired: 2 in, 2 out]
            n206 = case shown="True" w502 {
              frame False {
              }
              frame True {
                n207 = property on="Temp Chart" class="WFChart (strict)"("History Data"=dbl[] []) -> ()  [unwired: 2 in, 2 out]
              }
            }
          }
          event "StopProgram": Value Change {
            n208 = event-data() -> ()  [unwired: 1 in, 6 out]
          }
          event "Add Entry": Value Change {
            n209 = event-data() -> ()  [unwired: 1 in, 6 out]
            n210 = call "TableEntry.vi"("error in (no error)"=w527) -> ("error out"=w523:errorcluster, "Dwell Time @ SP (sec) 2"=w524:u32, "Cooling rate (°C/min) 2"=w525:dbl, "SP (°C) 2"=w526:dbl, "Add Entry Pressed?"=w528:bool)  [unwired: 6 in]
            n211 = case shown="True" w528 {
              tunnel: w526 -> [_ w537]
              tunnel: w525 -> [_ w536]
              tunnel: w524 -> [_ w535]
              tunnel: w523 -> [w530 w534]
              tunnel: [w530 w531] -> w522
              tunnel: w520 -> [w529 w533]
              tunnel: [w529 w532] -> w521
              frame False {
              }
              frame True {
                n212 = call "AddEntry2Table.vi"("Dwell Time @ SP (sec)"=w535, "error in (no error)"=w534, "Cooling rate (°C/min)"=w536, "SP (°C)"=w537, "RampProgramModel in"=w533) -> ("error out"=w531:errorcluster, "RampProgramModel out"=w532:refnum<class "RampProgramModel.lvclass">)  [unwired: 5 in]
              }
            }
          }
          event "Clear Table": Value Change {
            n213 = event-data() -> ()  [unwired: 1 in, 6 out]
            n214 = call "WriteRampTable.vi"("error in (no error)"=w544, "RampFromFile"=dbl[][] [], "RampProgramModel in"=w545) -> ("error out"=w543:errorcluster, "RampProgramModel out"=w542:refnum<class "RampProgramModel.lvclass">)  [unwired: 7 in]
          }
        }
        n215 = local read "stop"() -> (w248:bool)
        "Ramp Controller" <- w245
      }
    }
    frame Error {
    }
  }
  n216 = while {
    shift-right: [w555] -> _
    shift-left: AVI_recoder_state."Stop" -> [w560]
    tunnel: w25 -> [w559]
    tunnel: "error in (no error) 2" -> [w558]
    tunnel: [w557] -> w9
    shift-right: [w553] -> _
    shift-left: AVI_recoder_state."Stop" -> [w554]
    shift-right: [w552] -> _
    shift-left: T6 refnum ("AVI Refnum") -> [w551]
    shift-right: [w550] -> _
    shift-left: TRUE -> [w550]
    shift-right: [w548] -> _
    shift-left: w7 -> [w549]
    stop <- w561 continue-if-true
    n217 = event shown="[0] Timeout" {
      selector: _ -> [_ _ _ _ _]
      dyn-events: _ -> [_ _ _ _ _]
      timeout: w559 -> [_ _ _ _ _]
      tunnel: w560 -> [w574 w649 w664 w680 _]
      tunnel: w558 -> [w573 w651 w656 w678 w691]
      tunnel: [w572 w645 w655 w678 w687] -> w557
      tunnel: [w571 _ _ _ _] -> w556
      tunnel: [w570 w649 w665 w681 AVI_recoder_state."Stop"] -> w555
      tunnel: w554 -> [w569 w648 _ _ w704]
      tunnel: [w568 w648 w664 w680 w704] -> w553
      tunnel: [w567 w650 w663 w679 w703] -> w552
      tunnel: w551 -> [w566 w650 w663 w679 w703]
      tunnel: w549 -> [w565 w636 w654 w677 w686]
      tunnel: [w564 w636 w654 w677 w686] -> w548
      event Timeout {
        n218 = event-data() -> ()  [unwired: 1 in, 3 out]
        n219 = case shown="\"Stop\"" w574 {
          selector: w574 -> [w587 w592 w609 w634]
          tunnel: [w585 w594 w597 w630] -> w572
          tunnel: w573 -> [w577 w594 w611 w631]
          tunnel: [w585 w594 w598 w630] -> w571
          tunnel: [w587 w592 w609 AVI_recoder_state."Record"] -> w570
          tunnel: w569 -> [_ _ w608 _]
          tunnel: [w587 w592 w609 w634] -> w568
          tunnel: [w588 w593 T6 refnum ("AVI Refnum") w624] -> w567
          tunnel: w566 -> [w589 w593 w612 _]
          tunnel: w565 -> [w584 w590 w595 _]
          tunnel: [w583 w590 w595 w618] -> w564
          frame "Record", Default {
            (unwired) "%c" ("time format string (%c)")
            n220 = local read "Temp String (C)"() -> (w582:string)
            n221 = Format Date/Time String(time format string (%c)="%d/%%m/%Y %H:%M:%S%2u") -> (date/time string=w580:string)  [unwired: 2 in]
            n222 = call "Image-GFV.vi"("error in (no error)"=w577, "Image GFV Enum"=ImageEnum4GFV."Read") -> ("error out"=w576:errorcluster, "Output Image"=w575:T2)  [unwired: 8 in]
            n223 = Bundle("date/time string"=w580, "Temp String (C)"=w582) -> (w581:T12)  [unwired: 1 in]
            n224 = Build Array (concatenate)(w584, w581) -> (w583:T5)
            n225 = local write "Status"("Recording" ("Recorder Status")) -> ()
            n226 = call "IMAQ AVI2 Write Frame"("error in (no error)"=w576, "Image"=w575, "AVI Refnum"=w589) -> ("error out"=w585:errorcluster, "AVI Refnum (duplicate)"=w588:T6)  [unwired: 6 in, 1 out]
          }
          frame "Pause" {
            n227 = local write "Status"("Pause" ("Recorder Status")) -> ()
          }
          frame "Stop" {
            n228 = local read "Experiment Name"() -> (w605:string)
            n229 = Equal?(x=w609, y=w608) -> (x = y?=w607:bool)
            n230 = local read "File Path"() -> (w606:path)
            n231 = case shown="True" w607 {
              tunnel: w612 -> [w615 _]
              tunnel: w611 -> [w614 w616]
              tunnel: [w613 w616] -> w598
              frame False {
                n232 = call "IMAQ AVI2 Close"("error in (no error)"=w614, "AVI Refnum"=w615) -> ("error out"=w613:errorcluster)  [unwired: 9 in]
              }
              frame True {
              }
            }
            n233 = Empty String/Path?(string/path=w606) -> (empty?=w603:bool)
            n234 = Empty String/Path?(string/path=w605) -> (empty?=w604:bool)
            n235 = Or(x=w603, y=w604) -> (x .or. y?=w602:bool)
            n236 = Select(t=T4."Disabled and Grayed Out" ("Disabled"), s=w602, f=T4."Enabled" ("Disabled")) -> (s? t:f=w596:T4)
            n237 = property on="Record" class="Bool (strict)"(error in=w598, "DisabledEnum"=w596) -> (error out=w597:errorcluster)  [unwired: 1 in, 1 out]
            "Status" <- "Stop" ("Recorder Status")
          }
          frame "Init" {
            w618 = T5 []  # Date and Temp Cluster
            # "Create a file"
            n238 = call "IMAQ AVI2 Get Codec Names"() -> ("Codec Names"=w633:string[])  [unwired: 10 in, 1 out]
            n239 = local read "Experiment Name"() -> (w627:string)
            n240 = local read "File Path"() -> (w628:path)
            n241 = Index Array(array=w633, index="index 2") -> (element=w629:string)
            "Codec Type" <- w629
            n242 = Format Date/Time String(time format string (%c)="%d_%m_%Y-%H_%M_%S") -> (date/time string=w620:string)  [unwired: 2 in]
            n243 = Concatenate Strings(w627, "-" ("string"), w620, ".avi" ("string")) -> (w626:string)
            n244 = Build Path(base path=w628, name or relative path=w626) -> (appended path=w625:path)
            "Full avi Path and Name" <- w625
            n245 = call "IMAQ AVI2 Create"("error in (no error)"=w631, "Codec"=w629, "Frames Per Second"=u32 1, "AVI Path"=w625) -> ("error out"=w630:errorcluster, "AVI Refnum"=w624:T6)  [unwired: 6 in]
            n246 = local write "Status"("Init" ("Recorder Status")) -> ()
          }
        }
      }
      event "TakeRefImage": Value Change {
        n247 = event-data() -> ()  [unwired: 1 in, 6 out]
        n248 = call "Image-GFV.vi"("error in (no error)"=w651, "Image GFV Enum"=ImageEnum4GFV."Read") -> ("error out"=w646:errorcluster, "Output Image"=w647:T2)  [unwired: 8 in]
        "Reference Image" <- w647
        n249 = local read "Experiment Name"() -> (w643:string)
        n250 = local read "File Path"() -> (w644:path)
        n251 = Format Date/Time String(time format string (%c)="%d_%m_%Y-%H_%M_%S") -> (date/time string=w639:string)  [unwired: 2 in]
        n252 = Concatenate Strings(w643, "-" ("string"), w639, ".png" ("string")) -> (w642:string)
        n253 = Build Path(base path=w644, name or relative path=w642) -> (appended path=w638:path)
        n254 = call-poly "IMAQ Write File 2"("error in (no error)"=w646, "File Path"=w638, "Image"=w647) -> ("error out"=w645:errorcluster)  [unwired: 7 in, 1 out]
      }
      event "Record": Value Change {
        n255 = event-data() -> ()  [unwired: 1 in, 6 out]
        n256 = local read "Experiment Name"() -> (w661:string)
        n257 = local read "File Path"() -> (w662:path)
        n258 = local write "Record"(FALSE ("Record")) -> ()
        n259 = Empty String/Path?(string/path=w662) -> (empty?=w659:bool)
        n260 = Empty String/Path?(string/path=w661) -> (empty?=w660:bool)
        n261 = Or(x=w659, y=w660) -> (x .or. y?=w658:bool)
        n262 = Not(x=w658) -> (.not. x?=w657:bool)
        n263 = case shown="True" w657 {
          tunnel: [w667 w674] -> w665
          tunnel: w664 -> [w667 w673]
          tunnel: w656 -> [w666 w669]
          tunnel: [w666 w668] -> w655
          frame False {
          }
          frame True {
            n264 = property on="NewExperiment" class="Bool"(error in=w669, "DisabledEnum"=T4."Disabled and Grayed Out" ("Disabled")) -> (error out=w668:errorcluster)  [unwired: 1 in, 1 out]
            n265 = Equal?(x=w673, y=AVI_recoder_state."Stop") -> (x = y?=w671:bool)
            n266 = Select(t=AVI_recoder_state."Init", s=w671, f=AVI_recoder_state."Record") -> (s? t:f=w674:T7)
          }
        }
      }
      event "Pause": Value Change {
        n267 = event-data() -> ()  [unwired: 1 in, 6 out]
        n268 = Equal?(x=w680, y=AVI_recoder_state."Record") -> (x = y?=w683:bool)
        n269 = Select(t=AVI_recoder_state."Pause", s=w683, f=w680) -> (s? t:f=w681:T7)
      }
      event "Stop": Value Change {
        # "Save Ascii file with Experiments details"
        n270 = event-data() -> ()  [unwired: 1 in, 6 out]
        n271 = local read "Experiment Name"() -> (w692:string)
        n272 = local read "Goal"() -> (w693:string)
        n273 = local read "File Path"() -> (w696:path)
        n274 = local read "Ramp Program Table"() -> (w697:string[][])
        n275 = local read "Full avi Path and Name"() -> (w701:path)
        n276 = property on="Mag" class="Enum (strict)"() -> ("RingText.Text"=w700:string)  [unwired: 2 in, 2 out]
        n277 = local write "Stop"(FALSE ("Stop")) -> ()
        n278 = local read "Cycles"() -> (w699:u32)
        n279 = Path To String(path=w696) -> (string=w695:string)
        n280 = Number To Decimal String(number=w699) -> (decimal integer string=w698:string)  [unwired: 1 in]
        n281 = Bundle By Name(cluster=T11 {"Experiment Name"="", "Goal"="", "Remarks"="", "File Path"="", "Mag"="", "Repeat Program Number"="", "Full avi Path and Name"=path "", "Ramp Table "=[], "Date and Time"=[]} ("Ascii Experiment Data"), "Experiment Name"=w692, "Goal"=w693, "Remarks"="Remarks", "File Path"=w695, "Ramp Table"=w697, "Repeat Program Number"=w698, "Mag"=w700, "Full avi Path and Name"=w701, "Date and Time"=w686) -> (w690:T11)
        n282 = call "SaveExperimentDataToAsciiFile.vi"("error in (no error)"=w691, "Ascii Experiment Data"=w690) -> ("error out"=w688:errorcluster)  [unwired: 9 in]
        n283 = property on="NewExperiment" class="Bool"(error in=w688, "DisabledEnum"=T4."Enabled" ("Disabled")) -> (error out=w687:errorcluster)  [unwired: 1 in, 1 out]
      }
    }
    n284 = Unbundle By Name(w556) -> ("status"=w562:bool)
    n285 = local read "stop"() -> (w563:bool)
    n286 = Not Or(1:w563, 2:w562) -> (0:w561:bool)
    "Video Recorder" <- w550
  }
  n287 = call "IMAQ Create"("Image Name"="Grab and Save to AVI Acq", "error in (no error)"=w42) -> ("New Image"=w41:T2, "error out"=w35:errorcluster)  [unwired: 2 in, 1 out]
  n288 = call "Image-GFV.vi"("error in (no error)"=w35, "Image GFV Enum"=ImageEnum4GFV."Init") -> ("error out"=w34:errorcluster)  [unwired: 8 in, 1 out]
  n289 = while {
    tunnel: w6 -> [w759]
    tunnel: w34 -> [w758]
    tunnel: [w737] -> w38
    tunnel: [w736] -> w37
    shift-right: [w743] -> _
    shift-left: TRUE -> [w743]
    shift-right: ["High Resolution"] -> _
    shift-left: FALSE ("High Resolution") -> [w739]
    shift-right: [w735] -> w40
    shift-left: w41 -> [w734]
    shift-right: [w724] -> _
    shift-left: 0.0 ("Shutter (1-4095)") -> [w730]
    shift-right: [w725] -> _
    shift-left: 0.0 ("Gain (0-570)") -> [w729]
    i -> [w717]
    stop <- w755 continue-if-true
    # "Changing Exposure and Gain"
    # "For Changing Resolution"
    n290 = local read "Experiment Name"() -> (w744:string)
    n291 = Wait (ms)(milliseconds to wait=u32 10) -> ()  [unwired: 1 out]
    n292 = local read "Status of Temperature Controller"() -> (w749:string)
    n293 = property on="Cooling Rate (°C/min)" class="DigNum (strict)"() -> ("Value"=w747:dbl)  [unwired: 2 in, 2 out]
    n294 = local read "Setpoint (°C)"() -> (w742:dbl)
    n295 = local read "Temp String (C)"() -> (w748:string)
    n296 = Number To Fractional String(number=w747, precision (6)=i16 2) -> (F-format string=w745:string)  [unwired: 2 in]
    n297 = Number To Fractional String(number=w742, precision (6)=i16 1) -> (F-format string=w741:string)  [unwired: 2 in]
    n298 = call "IMAQ AVI2 Open"("AVI File Path"=path "W:/Lior/Phyto_Rice_500C_tripleConcentration-26_02_2015-15_23_52.avi") -> ("error out"=w718:errorcluster, "AVI Refnum"=w720:T6)  [unwired: 9 in]
    n299 = Bundle By Name(cluster=T13 {"Status"="", "Experiment Name"="", "Current Temp (C)"="", "Set Point (C)"="", "Cooling Rate (C/min)"="", "Mag"=enum."20x_LM"} ("TextOnImage"), "Current Temp (C)"=w748, "Set Point (C)"=w741, "Status"=w749, "Mag"="Mag", "Experiment Name"=w744, "Cooling Rate (C/min)"=w745) -> (w750:T13)
    n300 = disable-structure shown="Enabled" {
      disable-tunnel: w759 -> [w778 w780]
      disable-tunnel: w758 -> [w777 w781]
      disable-tunnel: [w776 w779] -> w716
      disable-tunnel: [w775 w781] -> _
      disable-tunnel: w734 -> [w774 w779]
      disable-tunnel: [w773 w780] -> w733
      frame Disabled {
        n301 = call <vilib>:"IMAQdx Grab.vi"("error in"=w777, "Image In"=w774, "Session In"=w778) -> ("error out"=w775:errorcluster, "Image Out"=w776:T2, "Session Out"=w773:T3)  [unwired: 1 in, 5 out]
      }
      frame Enabled {
      }
    }
    n302 = call "IMAQ AVI2 Read Frame"("error in (no error)"=w718, "Frame Number"=w717, "Image"=w716, "AVI Refnum"=w720) -> ("Image Out"=w713:T2)  [unwired: 5 in, 2 out]
    n303 = call "AddText2Image.vi"("High Resolution"="High Resolution", "TextOnImage"=w750, "Input Image"=w713) -> ("error out"=w752:errorcluster, "Output Image"=w715:T2)  [unwired: 7 in]
    n304 = Unbundle By Name(w752) -> ("status"=w757:bool)
    n305 = call "Image-GFV.vi"("error in (no error)"=w752, "Input Image"=w715, "Image GFV Enum"=ImageEnum4GFV."Write") -> ("error out"=w714:errorcluster)  [unwired: 7 in, 1 out]
    n306 = local read "stop"() -> (w756:bool)
    n307 = case shown="True" "Enable Droplet Detection" {
      tunnel: w714 -> [w760 w770]
      tunnel: w713 -> [w761 w769]
      tunnel: [w761 w767] -> w711
      tunnel: [w760 w765] -> w709
      tunnel: "Mag" -> [_ w762]
      frame False {
      }
      frame True {
        n308 = call "DropDetectionForLinkam.vi"("Max(µm)"="Max(µm)", "Min(µm)"="Min(µm)", "error in"=w770, "Mag"=w762, "Minimum match score"=800.0, "Image in"=w769) -> ("error out"=w766:errorcluster, "Matches (pixel)"=w771:T14, "Image Out"=w768:T2)  [unwired: 1 in, 2 out]
        n309 = call "AddDropletDetectionOverlay2Image.vi"("error in (no error)"=w766, "Matches (pixel)"=w771, "Input Image"=w768) -> ("error out"=w765:errorcluster, "Output Image"=w767:T2)  [unwired: 7 in]
      }
    }
    n310 = local read "Status"() -> (w707:string)
    n311 = Not Or(1:w756, 2:w757) -> (0:w755:bool)
    n312 = call "AddRecordingOverlay2Image.vi"("error in (no error)"=w709, "Recording Status String"=w707, "Input Image"=w711) -> ("error out"=w712:errorcluster, "Output Image"=→"Image":T2)  [unwired: 7 in]
    n313 = Not Equal?(x=w730, y="Shutter (1-4095)") -> (x != y?=w732:bool)
    n314 = Not Equal?(x=w729, y="Gain (0-570)") -> (x != y?=w731:bool)
    n315 = Or(x=w732, y=w731) -> (x .or. y?=w728:bool)
    n316 = case shown="True" w728 {
      tunnel: w733 -> [w783 w790]
      tunnel: "Shutter (1-4095)" -> [_ w788]
      tunnel: "Gain (0-570)" -> [_ w787]
      tunnel: [w783 w786] -> w723
      tunnel: w712 -> [w782 w785]
      tunnel: [w782 w784] -> w722
      frame False {
      }
      frame True {
        n317 = property class="IMAQdx"(reference=w790, error in=w785, "ActiveAttribute"="CameraAttributes::Shutter::Value", "ValueDBL"=w788, "ActiveAttribute"="CameraAttributes::Gain::Value", "ValueDBL"=w787) -> (reference out=w786:T3, error out=w784:errorcluster)
      }
    }
    n318 = Not Equal?(x=w739, y="High Resolution") -> (x != y?=w738:bool)
    n319 = case shown="True" w738 {
      tunnel: w723 -> [w796 w819]
      tunnel: [w796 w810] -> w737
      tunnel: "High Resolution" -> [_ w809]
      tunnel: w722 -> [w794 w808]
      tunnel: [w794 w803] -> w736
      tunnel: w734 -> [w795 w806]
      tunnel: [w795 w798] -> w735
      tunnel: "Gain (0-570)" -> [w793 _]
      tunnel: "Shutter (1-4095)" -> [w792 _]
      tunnel: [w793 w797] -> w725
      tunnel: [w792 w797] -> w724
      frame False {
      }
      frame True {
        w797 = 0.0 ("Gain (0-570)")
        n320 = local read "Session In"() -> (w818:T3)
        n321 = call <vilib>:"IMAQdx Close Camera.vi"("error in"=w808, "Session In"=w819) -> ("error out"=w820:errorcluster)  [unwired: 9 out]
        n322 = call <vilib>:"IMAQdx Open Camera.vi"("error in"=w820, "Session In"=w818) -> ("error out"=w813:errorcluster, "Session Out"=w814:T3)  [unwired: 1 in, 7 out]
        n323 = Select(t=u32 15 ("f"), s=w809, f=u32 8) -> (s? t:f=w815:u32)
        n324 = property class="IMAQdx"(reference=w814, error in=w813, "VideoMode"=w815) -> (reference out=w812:T3, error out=w811:errorcluster)
        n325 = call <vilib>:"IMAQdx Configure Grab.vi"("error in"=w811, "Session In"=w812) -> ("error out"=w807:errorcluster, "Session Out"=w810:T3)  [unwired: 8 out]
        n326 = call "IMAQ Dispose"("Image"=w806, "error in (no error)"=w807) -> ("error out"=w801:errorcluster)  [unwired: 1 in, 3 out]
        n327 = call "Image-GFV.vi"("error in (no error)"=w801, "Image GFV Enum"=ImageEnum4GFV."Delete") -> ("error out"=w800:errorcluster)  [unwired: 8 in, 1 out]
        n328 = call "IMAQ Create"("Image Name"="New Grab", "error in (no error)"=w800) -> ("New Image"=w798:T2, "error out"=w804:errorcluster)  [unwired: 2 in, 1 out]
        n329 = call "Image-GFV.vi"("error in (no error)"=w804, "Image GFV Enum"=ImageEnum4GFV."Init") -> ("error out"=w803:errorcluster)  [unwired: 8 in, 1 out]
      }
    }
    "Video Grabber" <- w743
  }
  n330 = flat-sequence {
    tunnel: w13 -> [w821]
    tunnel: [w821] -> w12
    frame #0 {
      n331 = local write "Linkam Controller"(FALSE ("Linkam Controller")) -> ()
    }
  }
  n332 = flat-sequence {
    tunnel: w9 -> [w823]
    tunnel: [w823] -> w8
    frame #0 {
      n333 = local write "Video Recorder"(FALSE ("Video Recorder")) -> ()
    }
  }
  n334 = flat-sequence {
    tunnel: w15 -> [w825]
    tunnel: [w825] -> w14
    frame #0 {
      n335 = local write "Ramp Controller"(FALSE ("Ramp Controller")) -> ()
    }
  }
  n336 = VISA Close(VISA resource name=w50, error in (no error)=w12) -> (error out=w21:errorcluster)
  n337 = disable-structure shown="Disabled" {
    disable-tunnel: [w829 _] -> w39
    disable-tunnel: w38 -> [w828 _]
    disable-tunnel: w37 -> [w827 _]
    frame Disabled {
      n338 = call <vilib>:"IMAQdx Close Camera.vi"("error in"=w827, "Session In"=w828) -> ("error out"=w829:errorcluster)  [unwired: 9 out]
    }
    frame Enabled {
    }
  }
  n339 = Merge Errors(w8, w10, w21, w14) -> (w20:errorcluster)
  n340 = call "IMAQ Dispose"("Image"=w40, "error in (no error)"=w39) -> ("error out"=w11:errorcluster)  [unwired: 1 in, 3 out]
  n341 = flat-sequence {
    tunnel: w20 -> [w830]
    tunnel: [w830] -> w19
    frame #0 {
      n342 = local write "stop"(FALSE ("stop")) -> ()
    }
  }
  n343 = flat-sequence {
    tunnel: w11 -> [w832]
    tunnel: [w832] -> w10
    frame #0 {
      n344 = local write "Video Grabber"(FALSE ("Video Grabber")) -> ()
    }
  }
  n345 = call "Image-GFV.vi"("error in (no error)"=w19, "Image GFV Enum"=ImageEnum4GFV."Delete") -> ("error out"=w33:errorcluster)  [unwired: 8 in, 1 out]
  n346 = call <vilib>:"Simple Error Handler.vi"("error in (no error)"=w33) -> ()  [unwired: 2 in, 7 out]
